vi "Periodic Tasks.vi"(8 "error in":errorcluster) -> ()   [LabVIEW 2014]
doc: "This VI runs in parallel to other tasks. It can contain as many user-defined periodic loops as you need. These can carry out PID or other sorts of timed response."
uses:
  <vilib>/Rock Robotics/WPI/DriverStation/WPI_DriverStationRobotMode2.ctl
  <vilib>/Rock Robotics/WPI/Solenoid/WPI_SolenoidValue.ctl
  Robot Global Data.vi
  <vilib>/addons/control/pid/pid.llb/PID (DBL).vi
  <vilib>/Rock Robotics/WPI/Solenoid/WPI_SolenoidSetEnum.vi
  <vilib>/addons/control/pid/NI_PID_pid.lvlib
panel:
  out "Elevador":dbl
  # "3609.35"
  # "476.5"
  # "Direita -> 0.13202 Tick/cm"
  # "Esquerda -> -0.04186 Tick/cm"
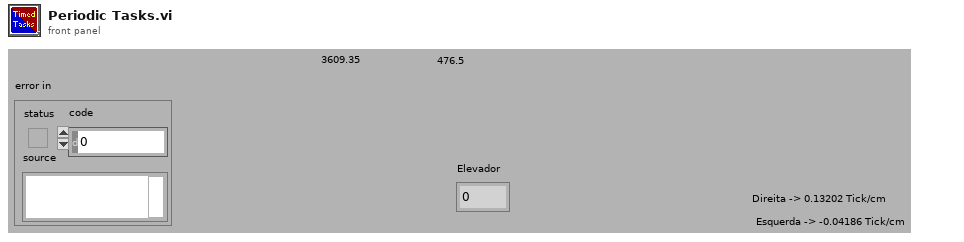
[diagram p1: front panel]
types:
  T1 = enum16{"Wait", "Empty state", "Get Bin", "Get Tote First", "Get Knocked Bin", "Close Gripper - Bin", "Close Gripper", "Carry Bin Mode", "Carry Tote Mode", "Get Tote", "Change Height", "Open Gripper", "Get to 0", "Release Pile"}
  T2 = enum16{"Espera o botão", "Bate", "Para", "Volta", ""}
  T3 = typedef "WPI_MotorControlDeviceRef.ctl" = cluster{"DeviceStatus":errorcluster, "Type":T4, "PWM":cluster{"Controller":T5, "PWM Channel":T6, "DeadBand":T7}, "CAN":cluster{"Device Number":u8, "Control Mode":T8, "Semaphore":T9, "Max Vout":dbl, "TalonSRX Control Mode":T10}, "Invert":bool, "TransformRef":T11, "InvTransformRef":T11}
  T4 = typedef "WPI_MotorControlType.ctl" = enum16{"PWM", "CAN", "CANTalonSRX"}
  T5 = typedef "FPGA_TypedefDigitalModule.ctl" = enum16{"Controller 1"}
  T6 = typedef "FPGA_DIOPWMChannel.ctl" = enum8{"PWM 0", "PWM 1", "PWM 2", "PWM 3", "PWM 4", "PWM 5", "PWM 6", "PWM 7", "PWM 8", "PWM 9", "PWM MXP 0", "PWM MXP 1", "PWM MXP 2", "PWM MXP 3", "PWM MXP 4", "PWM MXP 5", "PWM MXP 6", "PWM MXP 7", "PWM MXP 8", "PWM MXP 9", "Invalid"}
  T7 = typedef "WPI_PWMDeadband.ctl" = cluster{"Name":string, "maxPositivePwm":i32, "minPositivePwm":i32, "centerPwm":i32, "maxNegativePwm":i32, "minNegativePwm":i32, "angularRange":u16}
  T8 = typedef "WPI_CANJaguar_ControlMode.ctl" = enum8{"Percent VBus", "Current", "Speed", "Position", "Voltage"}
  T9 = typedef "Semaphore RefNum" = refnum<k1>
  T10 = typedef "WPI_CANTalonSRX_APIControlMode.ctl" = enum8{"Percent VBus", "Speed", "Position", "Slave", "Unchanged / Invalid"}
  T11 = typedef "WPI_PWMTransform_ConPane.ctl" = refnum<vi>
  T12 = typedef "WPI_DriverStationRobotMode2.ctl" = enum16{"Autonomous Disabled", "Autonomous Enabled", "Teleop Disabled", "Teleop Enabled", "Disconnected", "Finish", "Test Disabled", "Test Enabled", "Emergency Stopped"}
  T13 = typedef "WPI_SwitchDevRef.ctl" = cluster{"DevStatus":errorcluster, "DIO Channel":T14, "Controller":T5, "CntIndex":T15, "Normally Closed":bool}
  T14 = typedef "FPGA_DIOChannel.ctl" = enum8{"DIO 0", "DIO 1", "DIO 2", "DIO 3", "DIO 4", "DIO 5", "DIO 6", "DIO 7", "DIO 8", "DIO 9", "DIO MXP 0", "DIO MXP 1", "DIO MXP 2", "DIO MXP 3", "DIO MXP 4", "DIO MXP 5", "DIO MXP 6", "DIO MXP 7", "DIO MXP 8", "DIO MXP 9", "DIO MXP 10", "DIO MXP 11", "DIO MXP 12", "DIO MXP 13", "DIO MXP 14", "DIO MXP 15", "Invalid"}
  T15 = typedef "FPGA_CounterCtrSystemIndex.ctl" = enum8{"Ctr 0", "Ctr 1", "Ctr 2", "Ctr 3", "Ctr 4", "Ctr 5", "Ctr 6", "Ctr 7", "Invalid"}
  T16 = typedef "WPI_EncoderDevRef.ctl" = cluster{"DevStatus":errorcluster, "EncoderIndex":T17, "CounterIndex":T15, "DistancePerCount":dbl, "Decoding Type":T18}
  T17 = typedef "FPGA_EncoderIdx.ctl" = enum8{"Enc 0", "Enc 1", "Enc 2", "Enc 3", "Enc 4", "Enc 5", "Enc 6", "Enc 7", "Invalid"}
  T18 = typedef "WPI_EncoderType.ctl" = enum16{"1x", "2x", "4x"}
  T19 = typedef "WPI_AnalogChannelDevRef.ctl" = cluster{"DevStatus":errorcluster, "Controller":T20, "Analog Channel":T21}
  T20 = typedef "FPGA_TypedefAnalogModule.ctl" = enum16{"Controller 1"}
  T21 = typedef "FPGA_AIChannel.ctl" = enum8{"AI 0", "AI 1", "AI 2", "AI 3", "AI MXP 0", "AI MXP 1", "AI MXP 2", "AI MXP 3", "Invalid"}
  T22 = typedef "WPI_SolenoidDevRef.ctl" = cluster{"DevStatus":errorcluster, "Pneumatics Control Module":u8, "Forward Solenoid Channel":T23, "Reverse Solenoid Channel":T23}
  T23 = typedef "WPI_SolenoidChannel.ctl" = enum8{"Solenoid 0", "Solenoid 1", "Solenoid 2", "Solenoid 3", "Solenoid 4", "Solenoid 5", "Solenoid 6", "Solenoid 7", "Invalid"}
  T24 = cluster{"proportional gain (Kc)":dbl, "integral time (Ti, min)":dbl, "derivative time (Td, min)":dbl}
  T25 = typedef "WPI_SolenoidValue.ctl" = enum16{"Off", "On", "Forward", "Reverse"}
  T26 = enum16{"open", "replace", "create", "open or create", "replace or create", "replace or create with confirmation"}
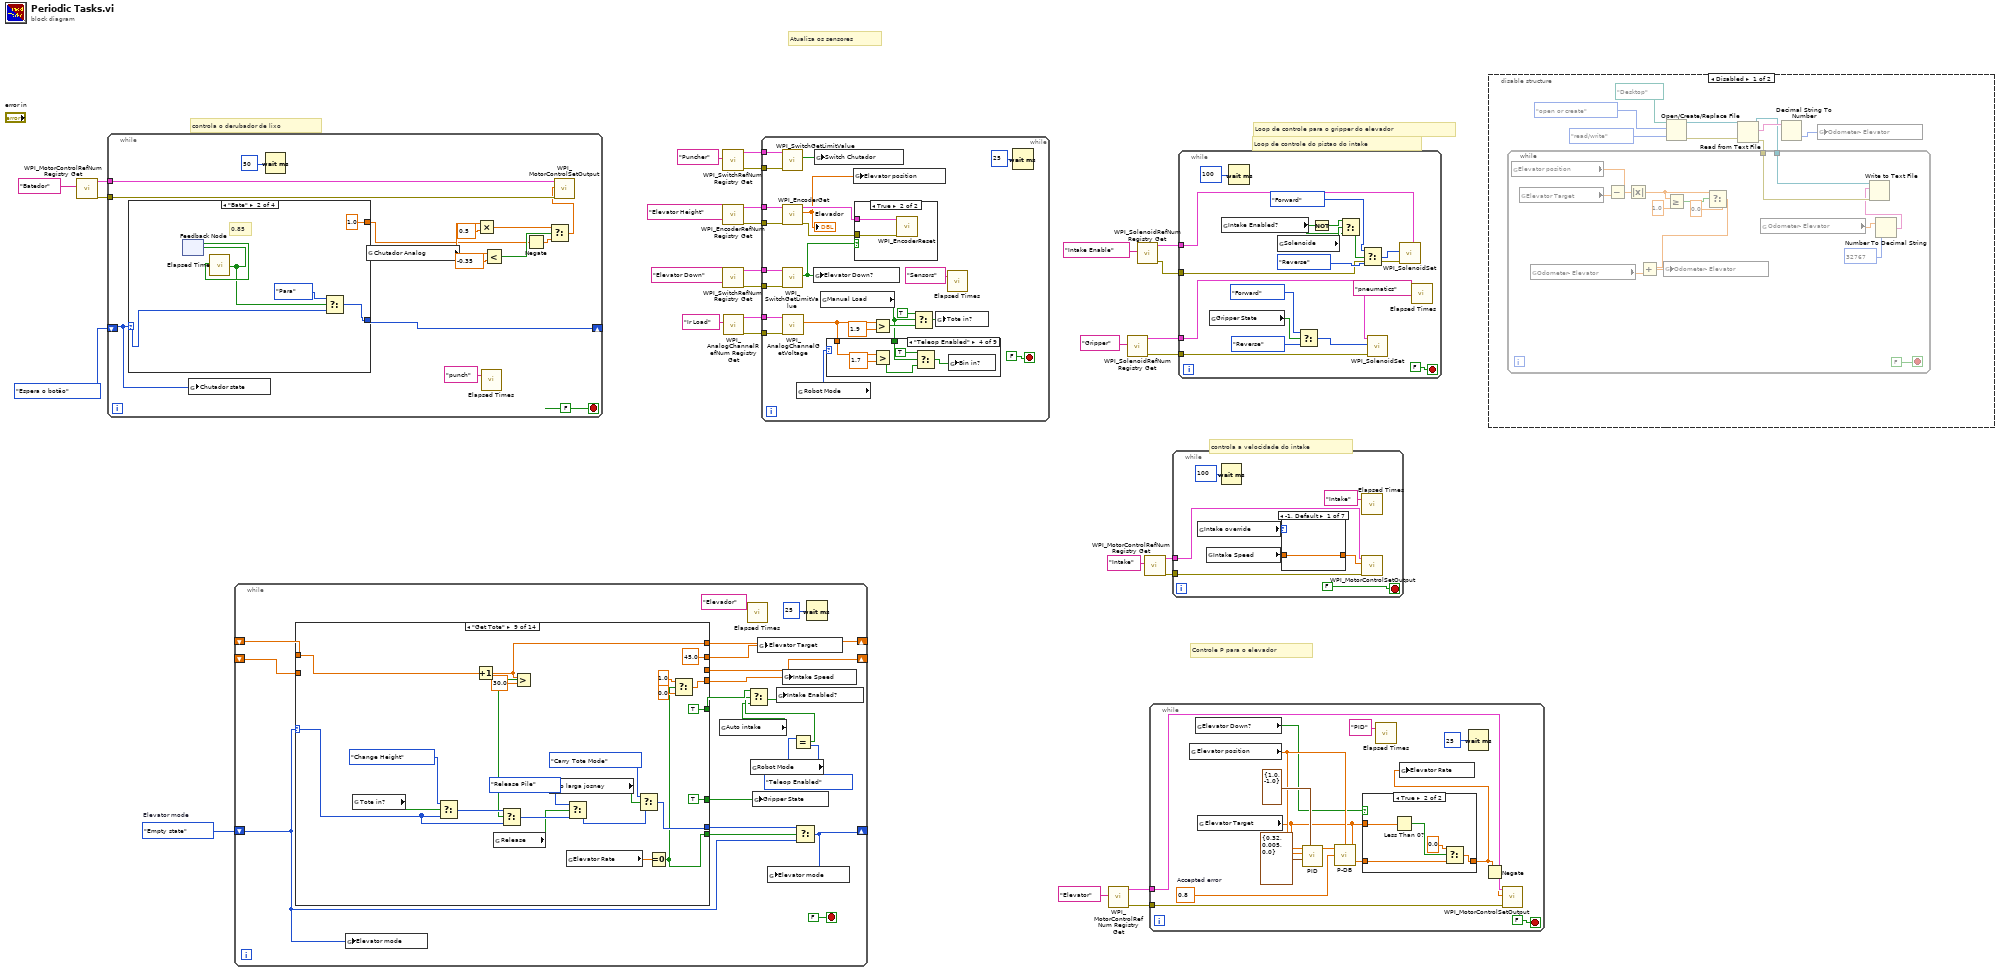
[diagram p0: block diagram]
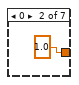
[diagram p4: hidden frame]
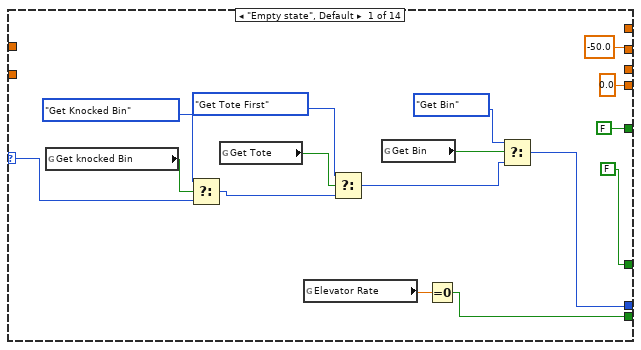
[diagram p10: hidden frame]
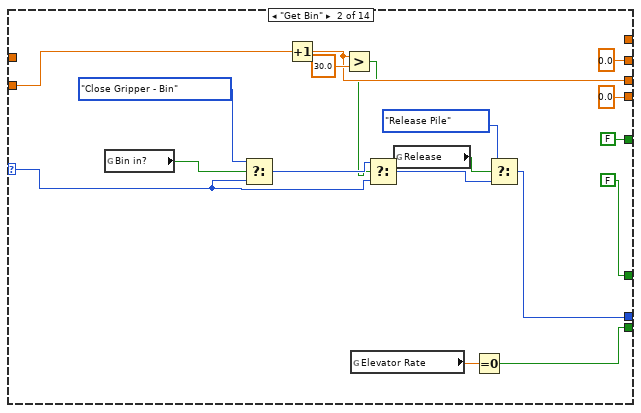
[diagram p11: hidden frame]
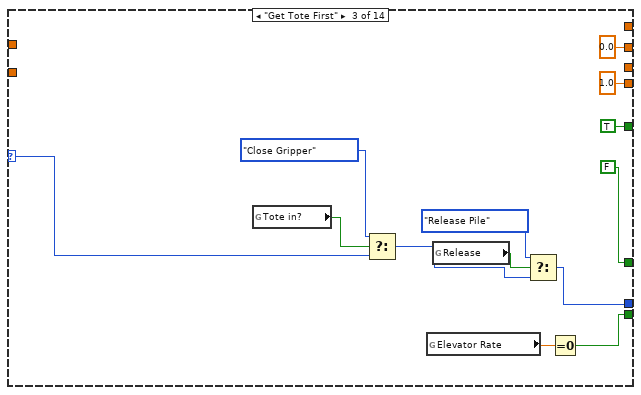
[diagram p12: hidden frame]
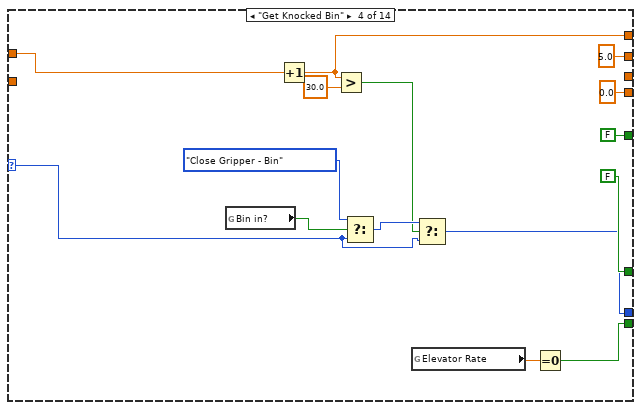
[diagram p13: hidden frame]
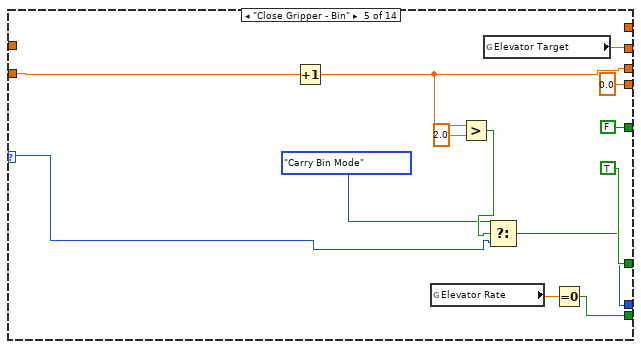
[diagram p14: hidden frame]
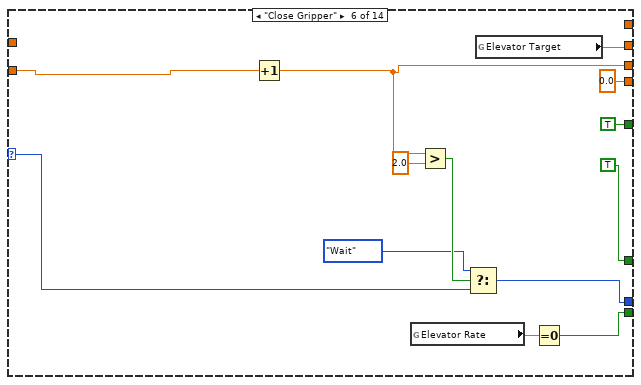
[diagram p15: hidden frame]
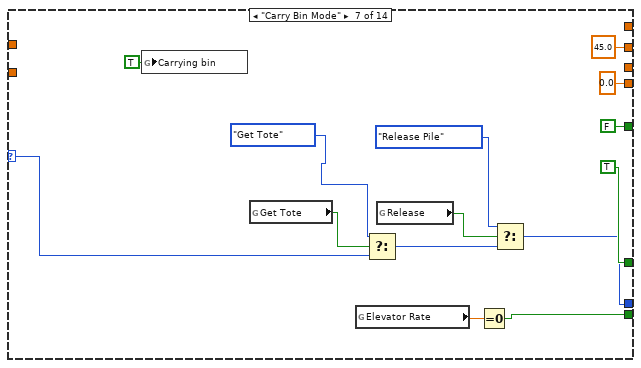
[diagram p16: hidden frame]
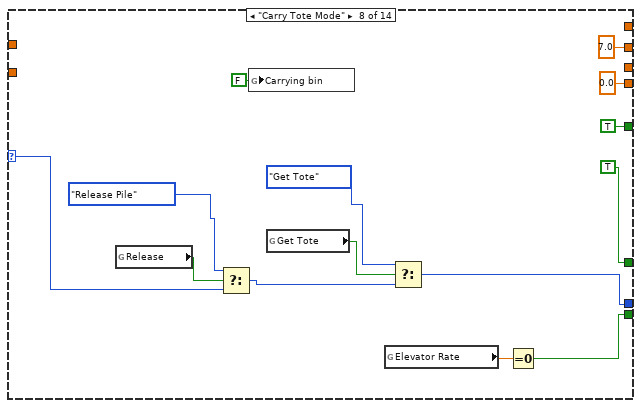
[diagram p17: hidden frame]
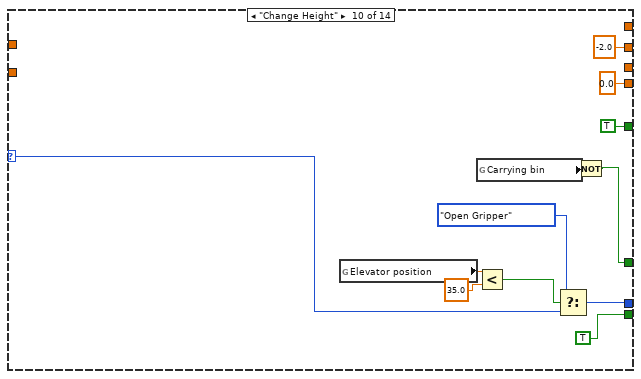
[diagram p18: hidden frame]
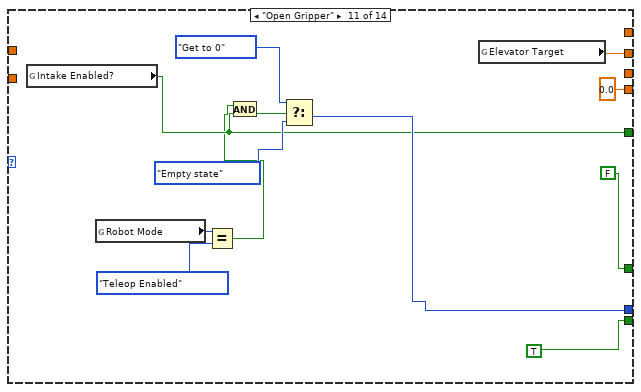
[diagram p19: hidden frame]
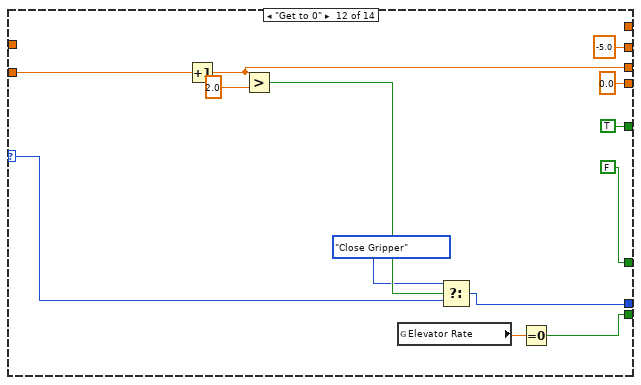
[diagram p20: hidden frame]
diagram:
  w1 = T1."Empty state"  # Elevator mode
  # "Controle P para o elevador"
  # "controla o derubador de lixo"
  # "Atualiza os sensores"
  # "controla a velocidade do intake"
  # "Loop de controle do pistao do intake"
  # "Loop de controle para o gripper do elevador"
  n1 = call <vilib>:"WPI_MotorControlRefNum Registry Get.vi"("refnum name"="Batedor") -> ("error out"=w26:errorcluster, "MotorControlDevRef"=w27:T3)  [unwired: 9 in]
  n2 = while {
    shift-right: [w43] -> _
    shift-left: T2."Espera o botão" -> [w30]
    tunnel: w27 -> [w42]
    tunnel: w26 -> [w41]
    stop <- FALSE stop-if-true
    n3 = case shown="\"Bate\"" w30 {
      selector: w30 -> [w50 w54 w60 w66]
      tunnel: [w47 w56 w62 w67] -> w43
      tunnel: [0.0 ("Output") 1.0 ("Output") 0.0 ("Output") -0.4 ("Output")] -> w34
      frame "Espera o botão", Default {
        # "Espera o botao ser ativado\npara derubar o lixo/caixa"
        n4 = global read "Robot Global Data.vi" "Chutador"() -> (w52:bool)
        n5 = global read "Robot Global Data.vi" "Chutador Volta"() -> (w45:bool)
        n6 = Select(t=T2."Bate", s=w52, f=w50) -> (s? t:f=w48:T2)
        n7 = Select(t=T2."Volta", s=w45, f=w48) -> (s? t:f=w47:T2)
      }
      frame "Bate" {
        # "0.85"
        n8 = feedback #1() -> (w57:bool)  [unwired: 1 in]
        n9 = call "Elapsed Time"("Reset"=w57) -> ("Time has Elapsed"=w53:bool)  [unwired: 11 in, 7 out]
        n10 = feedback-in #1(w53) -> ()
        n11 = Select(t=T2."Para", s=w53, f=w54) -> (s? t:f=w56:T2)
      }
      frame "Para" {
        # "Para o batedor por 300ms"
        n12 = feedback #2() -> (w63:bool)  [unwired: 1 in]
        n13 = call "Elapsed Time2"("Reset"=w63) -> ("Time has Elapsed"=w59:bool)  [unwired: 11 in, 7 out]
        n14 = feedback-in #2(w59) -> ()
        n15 = Select(t=T2."Volta", s=w59, f=w60) -> (s? t:f=w62:T2)
      }
      frame "Volta" {
        # "volta o batedor ate a limit switch"
        n16 = global read "Robot Global Data.vi" "Switch Chutador"() -> (w68:bool)
        n17 = Select(t=T2."Espera o botão", s=w68, f=w66) -> (s? t:f=w67:T2)
      }
    }
    n18 = global write "Robot Global Data.vi" "Chutador state"(w30) -> ()
    n19 = Wait (ms)(milliseconds to wait=u32 50) -> ()  [unwired: 1 out]
    n20 = global read "Robot Global Data.vi" "Chutador Analog"() -> (w37:dbl)
    n21 = Multiply(x=w37, y=0.5) -> (x*y=w35:dbl)
    n22 = call "Elapsed Times.vi"("Call Name"="punch") -> ()  [unwired: 2 in, 1 out]
    n23 = Less?(x=w37, y=-0.35) -> (x < y?=w38:bool)
    n24 = Negate(x=w34) -> (-x=w33:dbl)
    n25 = Select(t=w35, s=w38, f=w33) -> (s? t:f=w32:dbl)
    n26 = call <vilib>:"WPI_MotorControlSetOutput.vi"("error in (no error)"=w41, "Output"=w32, "MotorControlDevRef"=w42) -> ()  [unwired: 6 in, 3 out]
  }
  n27 = while {
    shift-right: [w77] -> _
    shift-left: w1 -> [w76]
    shift-right: [w82] -> _
    shift-left: _ -> [w83]
    shift-right: [w78] -> _
    shift-left: _ -> [w79]
    stop <- FALSE stop-if-true
    n28 = case shown="\"Get Tote\"" w76 {
      selector: w76 -> [w96 w115 w132 w144 w159 w172 w187 w199 w223 w233 _ w258 w274 w285]
      tunnel: [-50.0 ("Elevator position") 0.0 ("Elevator position") 0.0 ("Elevator position") 5.0 ("Elevator position") w161 w174 45.0 ("Elevator position") 7.0 ("Elevator position") 45.0 ("Elevator position") -2.0 ("Elevator position") w250 -5.0 ("Elevator position") -5.0 ("Elevator position") w289] -> w87
      tunnel: [FALSE FALSE TRUE FALSE FALSE TRUE FALSE TRUE TRUE TRUE w244 TRUE FALSE w287] -> w74
      tunnel: [w102 w109 w125 w142 w158 w173 w186 w201 w213 w237 w247 w256 w273 w286] -> w86
      tunnel: [0.0 ("Elevator position") 0.0 ("Elevator position") 1.0 ("Elevator position") 0.0 ("Elevator position") 0.0 ("Elevator position") 0.0 ("Elevator position") 0.0 ("Elevator position") 0.0 ("Elevator position") w209 0.0 ("Elevator position") 0.0 ("Elevator position") 0.0 ("Elevator position") 0.0 ("Elevator position") w288] -> w85
      tunnel: [FALSE FALSE FALSE FALSE TRUE TRUE TRUE TRUE TRUE ("Gripper State") w229 FALSE FALSE w266 w283] -> w84
      tunnel: w83 -> [_ w118 _ _ w153 w165 _ _ _ _ _ w261 _ _]
      tunnel: [_ w117 _ _ w156 w169 _ _ _ _ _ w259 _ _] -> w82
      tunnel: [w93 w112 w129 w140 w154 w167 w181 w195 w206 TRUE TRUE w254 w269 TRUE] -> w81
      tunnel: w79 -> [_ _ _ w138 _ _ _ _ w219 _ _ _ _ w281]
      tunnel: [_ _ _ w137 _ _ _ _ w218 _ _ _ _ w280] -> w78
      frame "Empty state", Default {
        n29 = global read "Robot Global Data.vi" "Get knocked Bin"() -> (w97:bool)
        n30 = Select(t=T1."Get Knocked Bin" ("Elevator mode"), s=w97, f=w96) -> (s? t:f=w95:T1)
        n31 = global read "Robot Global Data.vi" "Get Tote"() -> (w100:bool)
        n32 = global read "Robot Global Data.vi" "Elevator Rate"() -> (w94:dbl)
        n33 = Select(t=T1."Get Tote First" ("Elevator mode"), s=w100, f=w95) -> (s? t:f=w101:T1)
        n34 = global read "Robot Global Data.vi" "Get Bin"() -> (w103:bool)
        n35 = Equal To 0?(x=w94) -> (x = 0?=w93:bool)
        n36 = Select(t=T1."Get Bin" ("Elevator mode"), s=w103, f=w101) -> (s? t:f=w102:T1)
      }
      frame "Get Bin" {
        n37 = global read "Robot Global Data.vi" "Bin in?"() -> (w110:bool)
        n38 = Select(t=T1."Close Gripper - Bin" ("Elevator mode"), s=w110, f=w115) -> (s? t:f=w116:T1)
        n39 = Increment(x=w118) -> (x+1=w117:dbl)
        n40 = Greater?(x=w117, y=30.0) -> (0:w114:bool)
        n41 = global read "Robot Global Data.vi" "Elevator Rate"() -> (w113:dbl)
        n42 = Select(t=w116, s=w114, f=w115) -> (s? t:f=w108:T1)
        n43 = global read "Robot Global Data.vi" "Release"() -> (w107:bool)
        n44 = Equal To 0?(x=w113) -> (x = 0?=w112:bool)
        n45 = Select(t=T1."Release Pile", s=w107, f=w108) -> (s? t:f=w109:T1)
      }
      frame "Get Tote First" {
        n46 = global read "Robot Global Data.vi" "Tote in?"() -> (w131:bool)
        n47 = Select(t=T1."Close Gripper" ("Elevator mode"), s=w131, f=w132) -> (s? t:f=w124:T1)
        n48 = global read "Robot Global Data.vi" "Elevator Rate"() -> (w130:dbl)
        n49 = global read "Robot Global Data.vi" "Release"() -> (w127:bool)
        n50 = Select(t=T1."Release Pile", s=w127, f=w124) -> (s? t:f=w125:T1)
        n51 = Equal To 0?(x=w130) -> (x = 0?=w129:bool)
      }
      frame "Get Knocked Bin" {
        n52 = global read "Robot Global Data.vi" "Bin in?"() -> (w147:bool)
        n53 = Increment(x=w138) -> (x+1=w137:dbl)
        n54 = Greater?(x=w137, y=30.0) -> (0:w143:bool)
        n55 = Select(t=T1."Close Gripper - Bin" ("Elevator mode"), s=w147, f=w144) -> (s? t:f=w145:T1)
        n56 = global read "Robot Global Data.vi" "Elevator Rate"() -> (w141:dbl)
        n57 = Select(t=w145, s=w143, f=w144) -> (s? t:f=w142:T1)
        n58 = Equal To 0?(x=w141) -> (x = 0?=w140:bool)
      }
      frame "Close Gripper - Bin" {
        n59 = Increment(x=w153) -> (x+1=w156:dbl)
        n60 = global read "Robot Global Data.vi" "Elevator Rate"() -> (w155:dbl)
        n61 = Greater?(x=w156, y=2.0) -> (0:w157:bool)
        n62 = global read "Robot Global Data.vi" "Elevator Target"() -> (w161:dbl)
        n63 = Select(t=T1."Carry Bin Mode" ("Elevator mode"), s=w157, f=w159) -> (s? t:f=w158:T1)
        n64 = Equal To 0?(x=w155) -> (x = 0?=w154:bool)
      }
      frame "Close Gripper" {
        n65 = Increment(x=w165) -> (x+1=w169:dbl)
        n66 = global read "Robot Global Data.vi" "Elevator Rate"() -> (w168:dbl)
        n67 = Greater?(x=w169, y=2.0) -> (0:w170:bool)
        n68 = Select(t=T1."Wait" ("Elevator mode"), s=w170, f=w172) -> (s? t:f=w173:T1)
        n69 = global read "Robot Global Data.vi" "Elevator Target"() -> (w174:dbl)
        n70 = Equal To 0?(x=w168) -> (x = 0?=w167:bool)
      }
      frame "Carry Bin Mode" {
        n71 = global write "Robot Global Data.vi" "Carrying bin"(TRUE ("Carrying bin")) -> ()
        n72 = global read "Robot Global Data.vi" "Get Tote"() -> (w184:bool)
        n73 = global read "Robot Global Data.vi" "Elevator Rate"() -> (w182:dbl)
        n74 = Select(t=T1."Get Tote" ("Elevator mode"), s=w184, f=w187) -> (s? t:f=w185:T1)
        n75 = global read "Robot Global Data.vi" "Release"() -> (w183:bool)
        n76 = Equal To 0?(x=w182) -> (x = 0?=w181:bool)
        n77 = Select(t=T1."Release Pile" ("Elevator mode"), s=w183, f=w185) -> (s? t:f=w186:T1)
      }
      frame "Carry Tote Mode" {
        n78 = global read "Robot Global Data.vi" "Release"() -> (w197:bool)
        n79 = Select(t=T1."Release Pile" ("Elevator mode"), s=w197, f=w199) -> (s? t:f=w200:T1)
        n80 = global write "Robot Global Data.vi" "Carrying bin"(FALSE ("Carrying bin")) -> ()
        n81 = global read "Robot Global Data.vi" "Get Tote"() -> (w198:bool)
        n82 = global read "Robot Global Data.vi" "Elevator Rate"() -> (w196:dbl)
        n83 = Select(t=T1."Get Tote" ("Elevator mode"), s=w198, f=w200) -> (s? t:f=w201:T1)
        n84 = Equal To 0?(x=w196) -> (x = 0?=w195:bool)
      }
      frame "Get Tote" {
        n85 = global read "Robot Global Data.vi" "Tote in?"() -> (w226:bool)
        n86 = Select(t=T1."Change Height" ("Elevator mode"), s=w226, f=w223) -> (s? t:f=w224:T1)
        n87 = Increment(x=w219) -> (x+1=w218:dbl)
        n88 = global read "Robot Global Data.vi" "Release"() -> (w214:bool)
        n89 = Greater?(x=w218, y=30.0) -> (0:w222:bool)
        n90 = Select(t=w224, s=w222, f=w223) -> (s? t:f=w216:T1)
        n91 = global read "Robot Global Data.vi" "Po larga josney"() -> (w210:bool)
        n92 = global read "Robot Global Data.vi" "Elevator Rate"() -> (w221:dbl)
        n93 = Select(t=T1."Release Pile", s=w214, f=w216) -> (s? t:f=w212:T1)
        n94 = Select(t=T1."Carry Tote Mode", s=w210, f=w212) -> (s? t:f=w213:T1)
        n95 = Equal To 0?(x=w221) -> (x = 0?=w206:bool)
        n96 = Select(t=1.0 ("Elevator position"), s=w206, f=0.0) -> (s? t:f=w209:dbl)
      }
      frame "Change Height" {
        n97 = global read "Robot Global Data.vi" "Elevator position"() -> (w236:dbl)
        n98 = global read "Robot Global Data.vi" "Carrying bin"() -> (w230:bool)
        n99 = Less?(x=w236, y=35.0) -> (x < y?=w234:bool)
        n100 = Select(t=T1."Open Gripper" ("Elevator mode"), s=w234, f=w233) -> (s? t:f=w237:T1)
        n101 = Not(x=w230) -> (.not. x?=w229:bool)
      }
      frame "Open Gripper" {
        n102 = global read "Robot Global Data.vi" "Intake Enabled?"() -> (w244:bool)
        n103 = global read "Robot Global Data.vi" "Robot Mode"() -> (w243:T12)
        n104 = Equal?(x=w243, y=WPI_DriverStationRobotMode2."Teleop Enabled") -> (x = y?=w241:bool)
        n105 = And(x=w241, y=w244) -> (x .and. y?=w245:bool)
        n106 = Select(t=T1."Get to 0" ("Elevator mode"), s=w245, f=T1."Empty state" ("Elevator mode")) -> (s? t:f=w247:T1)
        n107 = global read "Robot Global Data.vi" "Elevator Target"() -> (w250:dbl)
      }
      frame "Get to 0" {
        n108 = Increment(x=w261) -> (x+1=w259:dbl)
        n109 = Greater?(x=w259, y=2.0) -> (0:w257:bool)
        n110 = global read "Robot Global Data.vi" "Elevator Rate"() -> (w255:dbl)
        n111 = Select(t=T1."Close Gripper" ("Elevator mode"), s=w257, f=w258) -> (s? t:f=w256:T1)
        n112 = Equal To 0?(x=w255) -> (x = 0?=w254:bool)
      }
      frame "Release Pile" {
        n113 = feedback #3() -> (w271:bool)  [unwired: 1 in]
        n114 = call "Elapsed Time7"("Reset"=w271) -> ("Time has Elapsed"=w272:bool)  [unwired: 11 in, 7 out]
        n115 = feedback-in #3(w272) -> ()
        n116 = global read "Robot Global Data.vi" "Elevator Rate"() -> (w270:dbl)
        n117 = global read "Robot Global Data.vi" "Carrying bin"() -> (w267:bool)
        n118 = Equal To 0?(x=w270) -> (x = 0?=w269:bool)
        n119 = Select(t=T1."Open Gripper" ("Elevator mode"), s=w271, f=w274) -> (s? t:f=w273:T1)
        n120 = Not(x=w267) -> (.not. x?=w266:bool)
      }
      frame "Wait" {
        n121 = Increment(x=w281) -> (x+1=w280:dbl)
        n122 = Greater?(x=w280, y=16.0) -> (0:w278:bool)
        n123 = global read "Robot Global Data.vi" "Elevator Target"() -> (w289:dbl)
        n124 = global read "Robot Global Data.vi" "Intake Enabled?"() -> (w287:bool)
        n125 = global read "Robot Global Data.vi" "Intake Speed"() -> (w288:dbl)
        n126 = global read "Robot Global Data.vi" "Gripper State"() -> (w283:bool)
        n127 = Select(t=T1."Carry Tote Mode" ("Elevator mode"), s=w278, f=w285) -> (s? t:f=w286:T1)
      }
    }
    n128 = global write "Robot Global Data.vi" "Elevator mode"(w76) -> ()
    n129 = global read "Robot Global Data.vi" "Auto intake"() -> (w70:bool)
    n130 = call "Elapsed Times.vi"("Call Name"="Elevador") -> ()  [unwired: 2 in, 1 out]
    n131 = global read "Robot Global Data.vi" "Robot Mode"() -> (w73:T12)
    n132 = global write "Robot Global Data.vi" "Gripper State"(w84) -> ()
    n133 = global write "Robot Global Data.vi" "Elevator Target"(w87) -> ()
    n134 = global write "Robot Global Data.vi" "Intake Speed"(w85) -> ()
    n135 = Equal?(x=WPI_DriverStationRobotMode2."Teleop Enabled", y=w73) -> (x = y?=w72:bool)
    n136 = Select(t=w74, s=w72, f=w70) -> (s? t:f=w75:bool)
    n137 = global write "Robot Global Data.vi" "Intake Enabled?"(w75) -> ()
    n138 = Select(t=w86, s=w81, f=w76) -> (s? t:f=w77:T1)
    n139 = global write "Robot Global Data.vi" "Elevator mode"(w77) -> ()
    n140 = Wait (ms)(milliseconds to wait=u32 25) -> ()  [unwired: 1 out]
  }
  n141 = call <vilib>:"WPI_SwitchRefNum Registry Get.vi"("refnum name"="Puncher") -> ("error out"=w23:errorcluster, "SwitchDevRef"=w24:T13)  [unwired: 9 in]
  n142 = call <vilib>:"WPI_EncoderRefNum Registry Get.vi"("refnum name"="Elevator Height") -> ("error out"=w15:errorcluster, "EncoderDevRef"=w16:T16)  [unwired: 9 in]
  n143 = call <vilib>:"WPI_SwitchRefNum Registry Get.vi"("refnum name"="Elevator Down") -> ("error out"=w19:errorcluster, "SwitchDevRef"=w18:T13)  [unwired: 9 in]
  n144 = call <vilib>:"WPI_AnalogChannelRefNum Registry Get.vi"("refnum name"="Ir Load") -> ("error out"=w22:errorcluster, "AIDeviceRef"=w21:T19)  [unwired: 9 in]
  n145 = while {
    tunnel: w24 -> [w309]
    tunnel: w23 -> [w308]
    tunnel: w21 -> [w302]
    tunnel: w22 -> [w303]
    tunnel: w18 -> [w306]
    tunnel: w19 -> [w307]
    tunnel: w16 -> [w305]
    tunnel: w15 -> [w304]
    stop <- FALSE stop-if-true
    n146 = call <vilib>:"WPI_SwitchGetLimitValue.vi"("error in (no error)"=w308, "SwitchDevRef"=w309) -> ("Switch Pressed"=w311:bool)  [unwired: 7 in, 2 out]
    n147 = call <vilib>:"WPI_EncoderGet.vi"("error in (no error)"=w304, "EncoderDevRef"=w305) -> ("error out"=w299:errorcluster, "Distance"=w298:dbl, "EncoderDevRef"=w300:T16)  [unwired: 4 in, 3 out]
    "Elevador" <- w298
    n148 = call <vilib>:"WPI_SwitchGetLimitValue.vi"("error in (no error)"=w307, "SwitchDevRef"=w306) -> ("Switch Pressed"=w301:bool)  [unwired: 7 in, 2 out]
    n149 = call <vilib>:"WPI_AnalogChannelGetVoltage.vi"("error in (no error)"=w303, "AIDeviceRef"=w302) -> ("Voltage"=w292:dbl)  [unwired: 7 in, 2 out]
    n150 = global read "Robot Global Data.vi" "Robot Mode"() -> (w291:T12)
    n151 = global write "Robot Global Data.vi" "Elevator Down?"(w301) -> ()
    n152 = global write "Robot Global Data.vi" "Switch Chutador"(w311) -> ()
    n153 = global read "Robot Global Data.vi" "Manual Load"() -> (w290:bool)
    n154 = case shown="\"Teleop Enabled\"" w291 {
      tunnel: w292 -> [w313 w316 _ w324 _ _ _ _ _]
      tunnel: w290 -> [_ _ _ w321 _ _ _ _ _]
      frame "Autonomous Disabled", Default {
        n155 = Greater?(x=w313, y=1.0) -> (0:w314:bool)
        n156 = global write "Robot Global Data.vi" "Bin in?"(w314) -> ()
      }
      frame "Autonomous Enabled" {
        n157 = Greater?(x=w316, y=1.0) -> (0:w317:bool)
        n158 = global write "Robot Global Data.vi" "Bin in?"(w317) -> ()
      }
      frame "Teleop Disabled" {
      }
      frame "Teleop Enabled" {
        n159 = Greater?(x=w324, y=1.7) -> (0:w320:bool)
        n160 = Select(t=TRUE, s=w321, f=w320) -> (s? t:f=w322:bool)
        n161 = global write "Robot Global Data.vi" "Bin in?"(w322) -> ()
      }
      frame "Disconnected" {
      }
      frame "Finish" {
      }
      frame "Test Disabled" {
      }
      frame "Test Enabled" {
      }
      frame "Emergency Stopped" {
      }
    }
    n162 = global write "Robot Global Data.vi" "Elevator position"(w298) -> ()
    n163 = case shown="True" w301 {
      tunnel: w300 -> [_ w326]
      tunnel: w299 -> [_ w325]
      frame False {
      }
      frame True {
        n164 = call <vilib>:"WPI_EncoderReset.vi"("error in (no error)"=w325, "EncoderDevRef"=w326) -> ()  [unwired: 8 in, 2 out]
      }
    }
    n165 = Greater?(x=w292, y=1.9) -> (0:w297:bool)
    n166 = Select(t=TRUE, s=w290, f=w297) -> (s? t:f=w296:bool)
    n167 = global write "Robot Global Data.vi" "Tote in?"(w296) -> ()
    n168 = call "Elapsed Times.vi"("Call Name"="Sensors") -> ()  [unwired: 2 in, 1 out]
    n169 = Wait (ms)(milliseconds to wait=u32 25) -> ()  [unwired: 1 out]
  }
  n170 = call <vilib>:"WPI_MotorControlRefNum Registry Get.vi"("refnum name"="Elevator") -> ("error out"=w5:errorcluster, "MotorControlDevRef"=w6:T3)  [unwired: 9 in]
  n171 = call <vilib>:"WPI_SolenoidRefNum Registry Get.vi"("refnum name"="Gripper") -> ("error out"=w2:errorcluster, "SolenoidDevRef"=w3:T22)  [unwired: 9 in]
  n172 = call <vilib>:"WPI_SolenoidRefNum Registry Get.vi"("refnum name"="Intake Enable") -> ("error out"=w11:errorcluster, "SolenoidDevRef"=w12:T22)  [unwired: 9 in]
  n173 = call <vilib>:"WPI_MotorControlRefNum Registry Get.vi"("refnum name"="Intake") -> ("error out"=w8:errorcluster, "MotorControlDevRef"=w9:T3)  [unwired: 9 in]
  n174 = while {
    tunnel: w6 -> [w340]
    tunnel: w5 -> [w339]
    stop <- FALSE stop-if-true
    w333 = 0.8  # Accepted error
    n175 = global read "Robot Global Data.vi" "Elevator position"() -> (w335:dbl)
    n176 = global read "Robot Global Data.vi" "Elevator Down?"() -> (w330:bool)
    n177 = global read "Robot Global Data.vi" "Elevator Target"() -> (w331:dbl)
    n178 = call-poly <vilib>:"PID.vi"("output range"=cluster{"output high":dbl, "output low":dbl} {"output high"=1.0, "output low"=-1.0}, "PID gains"=T24 {"proportional gain (Kc)"=0.32, "integral time (Ti, min)"=0.005, "derivative time (Td, min)"=0.0}, "process variable"=w335, "setpoint"=w331) -> ("output"=w334:dbl)  [unwired: 6 in, 1 out]
    n179 = call "P-DB.vi"("Setpoint"=w331, "Measured"=w335, "Accepted error"=w333, "Output"=w334) -> ("Output"=w332:dbl)  [unwired: 1 in]
    n180 = case shown="True" w330 {
      tunnel: w332 -> [w342 w344]
      tunnel: w331 -> [_ w347]
      tunnel: [w342 w343] -> w329
      frame False {
      }
      frame True {
        n181 = Less Than 0?(x=w347) -> (x < 0?=w346:bool)
        n182 = Select(t=0.0, s=w346, f=w344) -> (s? t:f=w343:dbl)
      }
    }
    n183 = call "Elapsed Times.vi"("Call Name"="PID") -> ()  [unwired: 2 in, 1 out]
    n184 = global write "Robot Global Data.vi" "Elevator Rate"(w329) -> ()
    n185 = Wait (ms)(milliseconds to wait=u32 25) -> ()  [unwired: 1 out]
    n186 = Negate(x=w329) -> (-x=w328:dbl)
    n187 = call <vilib>:"WPI_MotorControlSetOutput.vi"("error in (no error)"=w339, "Output"=w328, "MotorControlDevRef"=w340) -> ()  [unwired: 6 in, 3 out]
  }
  n188 = while {
    tunnel: w9 -> [w354]
    tunnel: w8 -> [w353]
    stop <- FALSE stop-if-true
    n189 = global read "Robot Global Data.vi" "Intake override"() -> (w350:dbl)
    n190 = global read "Robot Global Data.vi" "Intake Speed"() -> (w348:dbl)
    n191 = Wait (ms)(milliseconds to wait=u32 100) -> ()  [unwired: 1 out]
    n192 = case shown="-1, Default" w350 {
      tunnel: [w356 1.0 ("Intake Speed") _ _ _ _ _] -> w349
      tunnel: w348 -> [w356 _ _ _ _ _ _]
      frame -1, Default {
      }
      frame 0 {
      }
      frame 180 {
      }
      frame 270 {
      }
      frame 225 {
      }
      frame 135 {
      }
      frame 90 {
      }
    }
    n193 = call "Elapsed Times.vi"("Call Name"="Intake") -> ()  [unwired: 2 in, 1 out]
    n194 = call <vilib>:"WPI_MotorControlSetOutput.vi"("error in (no error)"=w353, "Output"=w349, "MotorControlDevRef"=w354) -> ()  [unwired: 6 in, 3 out]
  }
  n195 = while {
    tunnel: w12 -> [w372]
    tunnel: w11 -> [w371]
    tunnel: w3 -> [w363]
    tunnel: w2 -> [w364]
    stop <- FALSE stop-if-true
    n196 = global read "Robot Global Data.vi" "Gripper State"() -> (w368:bool)
    n197 = global read "Robot Global Data.vi" "Intake Enabled?"() -> (w360:bool)
    n198 = Wait (ms)(milliseconds to wait=u32 100) -> ()  [unwired: 1 out]
    n199 = global read "Robot Global Data.vi" "Solenoide"() -> (w362:bool)
    n200 = Select(t=WPI_SolenoidValue."Forward" ("Value"), s=w368, f=WPI_SolenoidValue."Reverse" ("Value")) -> (s? t:f=w367:T25)
    n201 = Not(x=w360) -> (.not. x?=w361:bool)
    n202 = Select(t=w361, s=w362, f=w360) -> (s? t:f=w359:bool)
    n203 = Select(t=WPI_SolenoidValue."Forward" ("Value"), s=w359, f=WPI_SolenoidValue."Reverse" ("Value")) -> (s? t:f=w375:T25)
    n204 = call-poly <vilib>:"WPI_SolenoidSet.vi"("error in (no error)"=w364, "Value"=w367, "SolenoidDevRef"=w363) -> ()  [unwired: 7 in, 2 out]
    n205 = call-poly <vilib>:"WPI_SolenoidSet.vi"("error in (no error)"=w371, "Value"=w375, "SolenoidDevRef"=w372) -> ()  [unwired: 7 in, 2 out]
    n206 = call "Elapsed Times.vi"("Call Name"="pneumatics") -> ()  [unwired: 2 in, 1 out]
  }
  n207 = disable-structure shown="Disabled" {
    frame Disabled {
      n208 = Open/Create/Replace File(file path (use dialog)=path "Desktop", operation (0:open)=T26."open or create", access (0:read/write)=enum16{"read/write", "read-only", "write-only"}."read/write") -> (refnum out=w378:refnum<file>, error out=w379:errorcluster)  [unwired: 3 in, 1 out]
      n209 = Read from Text File(file (use dialog)=w378, error in=w379) -> (refnum out=w377:refnum<file>, text=w381:string, error out=w376:errorcluster)  [unwired: 2 in, 1 out]
      n210 = while {
        tunnel: w377 -> [w389]
        tunnel: w376 -> [w388]
        stop <- FALSE stop-if-true
        n211 = global read "Robot Global Data.vi" "Elevator position"() -> (w398:dbl)
        n212 = global read "Robot Global Data.vi" "Elevator Target"() -> (w399:dbl)
        n213 = global read "Robot Global Data.vi" "Odometer- Elevator"() -> (w391:dbl)
        n214 = Subtract(x=w398, y=w399) -> (x-y=w397:dbl)
        n215 = Absolute Value(x=w397) -> (abs(x)=w393:dbl)
        n216 = Greater Or Equal?(x=w393, y=1.0) -> (x >= y?=w395:bool)
        n217 = Select(t=w393, s=w395, f=0.0) -> (s? t:f=w392:dbl)
        n218 = Add(x=w392, y=w391) -> (x+y=w390:dbl)
        n219 = global write "Robot Global Data.vi" "Odometer- Elevator"(w390) -> ()
        n220 = global read "Robot Global Data.vi" "Odometer- Elevator"() -> (w387:dbl)
        n221 = Number To Decimal String(number=w387, width (-)=i16 32767) -> (decimal integer string=w386:string)
        n222 = Write to Text File(file (use dialog)=w389, text=w386, error in=w388) -> ()  [unwired: 1 in, 3 out]
      }
      n223 = Decimal String To Number(string=w381) -> (number=w380:i32)  [unwired: 2 in, 1 out]
      n224 = global write "Robot Global Data.vi" "Odometer- Elevator"(w380) -> ()
    }
    frame Enabled {
    }
  }
